vi "Forward Kinematics.vi"(8 "Radii (ft)":T3 {"Right Back Position" format="%.2f"; "Right Front Position" format="%.2f"; "Left Back Position" format="%.2f"; "Left Front Position" format="%.2f"}, 10 "Steer Angles (degrees)":T2, 11 "Drive Velocities (ft/s)":T2) -> (3 "Robot Velocities (ft and deg)/s":T1)   [LabVIEW 2025]
uses:
  Type Definitions/Data/Pod Positions.ctl
  Type Definitions/Data/Robot Velocities.ctl
  <vilib>/Analysis/_algsub.llb/Real PseudoInverse Matrix.vi
  <vilib>/Analysis/baseanly.llb/A x Vector.vi
  <vilib>/Analysis/NI_AALPro.lvlib
  <vilib>/Analysis/NI_AALBase.lvlib
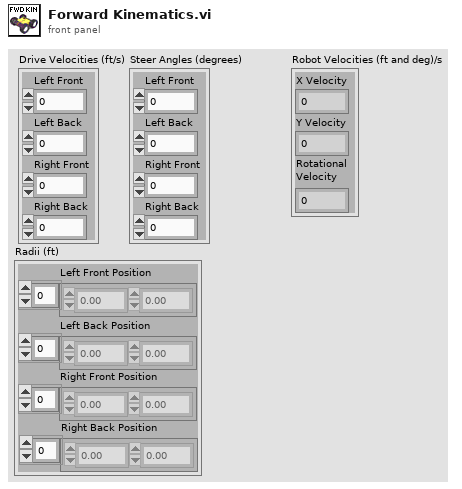
[diagram p1: front panel]
types:
  T1 = typedef "Robot Velocities.ctl" = cluster{"X Velocity":dbl, "Y Velocity":dbl, "Rotational \nVelocity":dbl}
  T2 = cluster{"Left Front":dbl, "Left Back":dbl, "Right Front":dbl, "Right Back":dbl}
  T3 = typedef "Pod Positions.ctl" = cluster{"Left Front Position":dbl[], "Left Back Position":dbl[], "Right Front Position":dbl[], "Right Back Position":dbl[]}
  T4 = typedef "NI_Matrix.lvlib/RealMatrix.ctl" = dbl[][]
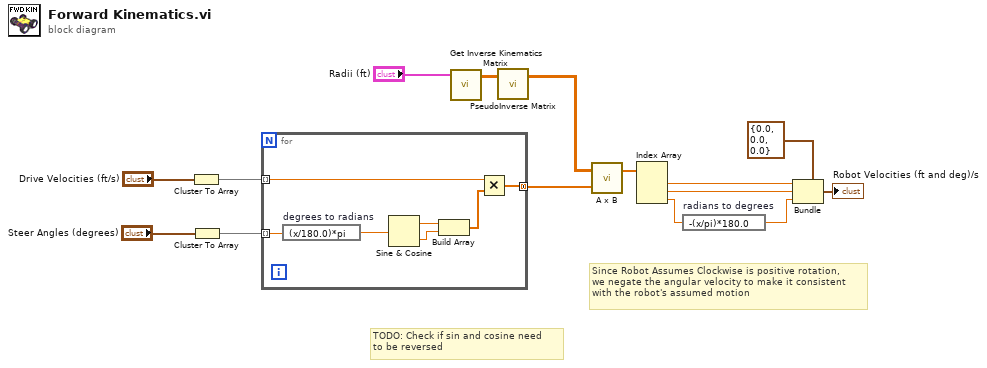
[diagram p0: block diagram]
diagram:
  # "TODO: Check if sin and cosine need\nto be reversed"
  # "Since Robot Assumes Clockwise is positive rotation,\nwe negate the angular velocity to make it consistent\nwith the robot's assumed motion"
  n1 = Cluster To Array(cluster="Drive Velocities (ft/s)") -> (array=w13:dbl[])
  n2 = Cluster To Array(cluster="Steer Angles (degrees)") -> (array=w12:dbl[])
  n3 = for {
    tunnel: w13 -> [w18] mode=indexing
    tunnel: w12 -> [w22] mode=indexing
    tunnel: [w16] -> w11 mode=concatenating
    n4 = expression code="(x/180.0)*pi" "degrees to radians"(w22) -> (w21:dbl)
    n5 = Sine & Cosine(0:w21) -> (1:w20:dbl, 2:w19:dbl)
    n6 = Build Array(w20, w19) -> (w17:dbl[])
    n7 = Multiply(x=w18, y=w17) -> (x*y=w16:dbl[])
  }
  n8 = call "Get Inverse Kinematics Matrix.vi"("Radii (ft)"="Radii (ft)") -> ("Real Matrix"=w14:T4)  [unwired: 10 in]
  n9 = call-poly <vilib>:"PseudoInverse Matrix.vi"("Input Matrix"=w14) -> ("PseudoInverse Matrix"=w10:T4)  [unwired: 1 in, 1 out]
  n10 = call-poly <vilib>:"A x B.vi"("Vector"=w11, "A"=w10) -> ("A x Vector"=w9:dbl[])  [unwired: 1 out]
  n11 = Index Array(array=w9) -> (element #1=w8:dbl, element #2=w7:dbl, element #3=w6:dbl)  [unwired: 3 in]
  n12 = expression code="-(x/pi)*180.0" "radians to degrees"(w6) -> (w5:dbl)
  n13 = Bundle(cluster=T1 {"X Velocity"=0.0, "Y Velocity"=0.0, "Rotational \nVelocity"=0.0} ("Robot Velocities (ft/s and deg/s)"), "X Velocity"=w8, "Y Velocity"=w7, "Rotational \nVelocity"=w5) -> (→"Robot Velocities (ft and deg)/s":T1)
